vi "XLP80_FGlob_DO.vi"(5 "Function (Set)":T1, 6 "Alarm":bool, 7 "PXI DO_Item":i32, 8 "err in":errorcluster caption="error", 10 "DXP Values IN":bool[](array[boolean]), 11 "DXP Value IN":bool) -> (0 "err out":errorcluster caption="error", 2 "DXP Values OUT":bool[](array[boolean]), 3 "DXP Value OUT":bool)   [LabVIEW 2021]
uses:
  1886_FGlob_TDefs_Enum_FGlobItems.ctl
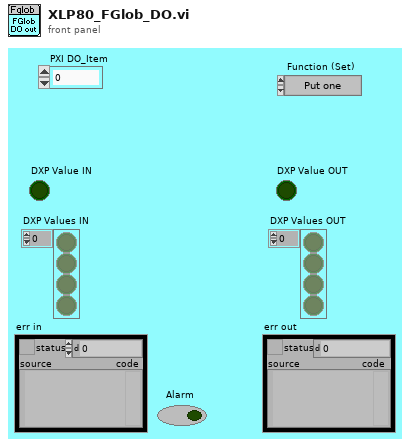
[diagram p1: front panel]
types:
  T1 = typedef "1886_FGlob_TDefs_Enum_FGlobItems.ctl" = enum16{"Put one", "Put all", "Recall one", "Recall all"}
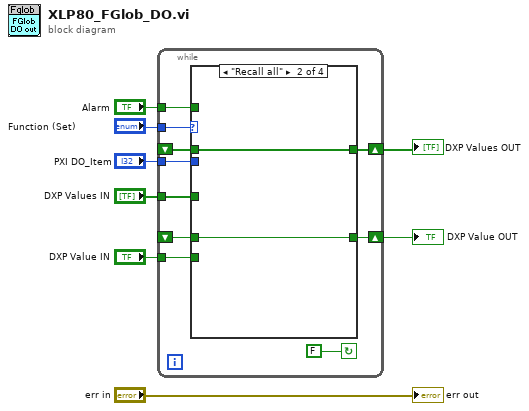
[diagram p0: block diagram]
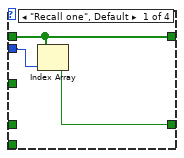
[diagram p2: hidden frame]
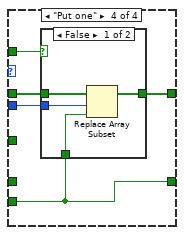
[diagram p5: hidden frame]
diagram:
  n1 = while {
    shift-right: [w16] -> w6
    shift-left: _ -> [w15]
    tunnel: "Function (Set)" -> [w17]
    tunnel: "PXI DO_Item" -> [w13]
    tunnel: "DXP Values IN" -> [w12]
    shift-right: [w14] -> w5
    shift-left: _ -> [w11]
    tunnel: "DXP Value IN" -> [w10]
    tunnel: "Alarm" -> [w9]
    stop <- FALSE continue-if-true
    n2 = case shown="\"Recall all\"" w17 {
      tunnel: [w21 w23 w25 w34] -> w16
      tunnel: w15 -> [w21 w23 w26 w35]
      tunnel: w13 -> [w20 _ _ w33]
      tunnel: [w19 w22 w28 w32] -> w14
      tunnel: w12 -> [_ _ w24 _]
      tunnel: w11 -> [_ w22 w28 _]
      tunnel: w10 -> [_ _ _ w32]
      tunnel: w9 -> [_ _ w27 w31]
      frame "Recall one", Default {
        n3 = Index Array(array=w21, index=w20) -> (element=w19:bool)
      }
      frame "Recall all" {
      }
      frame "Put all" {
        n4 = case shown="False" w27 {
          tunnel: [w29 w30] -> w25
          tunnel: w26 -> [_ w30]
          tunnel: w24 -> [w29 _]
          frame False {
          }
          frame True {
          }
        }
      }
      frame "Put one" {
        n5 = case shown="False" w31 {
          tunnel: w35 -> [w39 w40]
          tunnel: [w38 w40] -> w34
          tunnel: w33 -> [w37 _]
          tunnel: w32 -> [w36 _]
          frame False {
            n6 = Replace Array Subset(array=w39, new element=w36, index=w37) -> (w38:bool[])
          }
          frame True {
          }
        }
      }
    }
  }
  "DXP Values OUT" <- w6
  "DXP Value OUT" <- w5
  "err out" <- "err in"
